vi "CreateChannel.vi"(0 "task in":refnum<class "WaveformTask.lvclass">, 5 "Chan Name Array":string[](array[string]), 9 "instance":u8, 11 "error in":errorcluster) -> (4 "Task out":refnum<class "WaveformTask.lvclass">, 15 "error out":errorcluster)   [LabVIEW 2017, in "WaveformTask.lvclass"]
uses:
  WaveformTask.lvclass
  WaveformTask.lvclass/WaveformTask.ctl
  <instrlib>/_niInstr/FIFO Register Bus/v1/Host/niInstr FIFO Register Bus v1 Host.lvclass
  C:/Program Files (x86)/National Instruments/LabVIEW 2017/instr.lib/_niInstr/Instruction Framework/v1/Host/Instruction Target/niInstr Instruction Target v1 Host.lvclass
  <instrlib>/_niInstr/Instruction Framework/v1/Host/Subsystem Map/Private/Lookup Single Context.vi
  <instrlib>/_niInstr/Instruction Framework/v1/Host/Subsystem Map/niInstr Subsystem Map v1 Host.lvclass
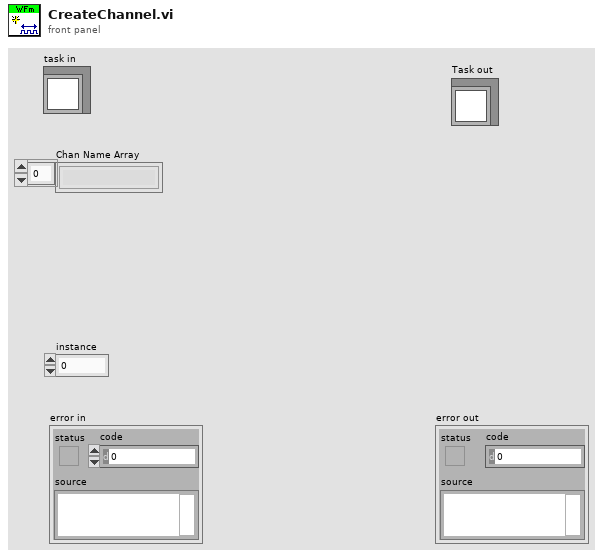
[diagram p1: front panel]
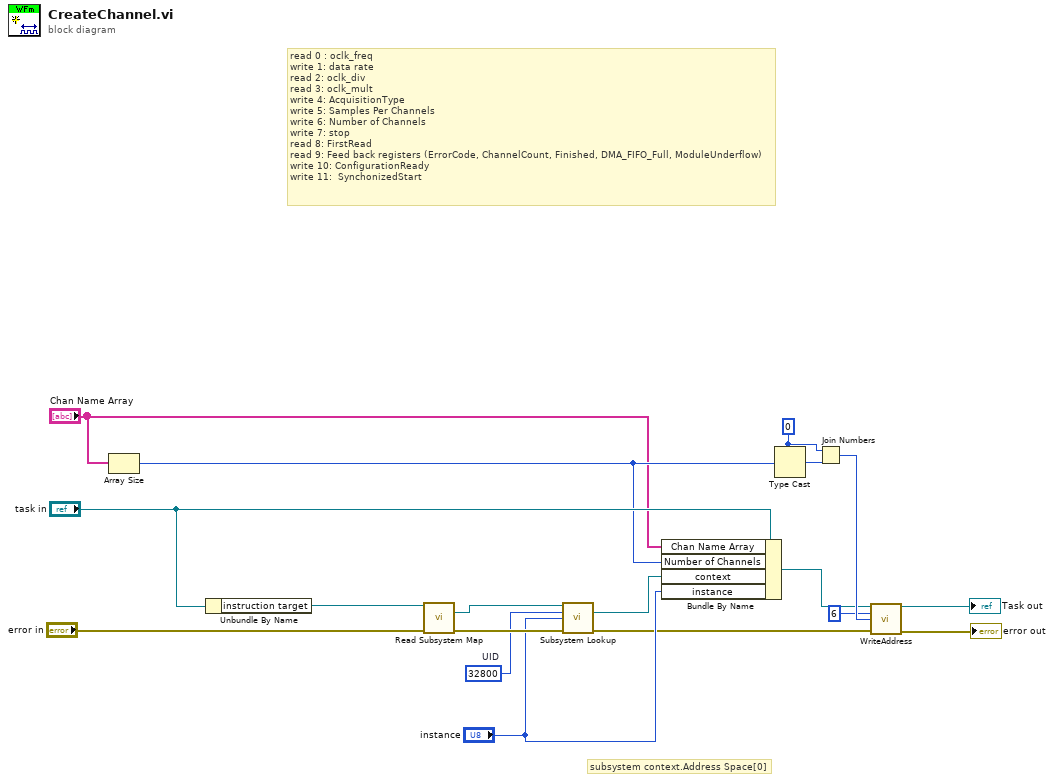
[diagram p0: block diagram]
diagram:
  w14 = u32 0
  w16 = u16 32800  # UID
  # "subsystem context.Address Space[0]"
  # "read 0 : oclk_freq\nwrite 1: data rate\nread 2: oclk_div\nread 3: oclk_mult\nwrite 4: AcquisitionType\nwrite 5: Samples Per Channels\nwrite 6: Number of Channels\nwrite 7: stop\nread 8: FirstRead\nread 9: Feed back registers (ErrorCode, ChannelCount, Finished, DMA_FIFO_Full, ModuleUnderflow)\nwrite 10: ConfigurationReady\nwrite 11:  SynchonizedStart"
  n1 = Array Size(array="Chan Name Array") -> (size(s)=w2:i32)
  n2 = Unbundle By Name("task in") -> ("instruction target"=w8:refnum<class "niInstr FIFO Register Bus v1 Host.lvclass">)
  n3 = call <instrlib>:"Read Subsystem Map.vi"("instruction target in"=w8, "error in"="error in") -> ("subsystem map"=w17:refnum<class "niInstr Subsystem Map v1 Host.lvclass">, "error out"=w18:errorcluster)  [unwired: 11 in, 1 out]
  n4 = call-poly <instrlib>:"Subsystem Lookup.vi"("subsystem map in"=w17, "UID"=w16, "instance"="instance", "error in"=w18) -> ("context"=w6:refnum<class "niInstr Instruction Framework Context v1 Host.lvclass">, "error out"=w3:errorcluster)  [unwired: 8 in, 2 out]
  n5 = Bundle By Name(cluster="task in", "Chan Name Array"="Chan Name Array", "Number of Channels"=w2, "context"=w6, "instance"="instance") -> (w4:refnum<class "WaveformTask.lvclass">)
  n6 = Type Cast(type=w14, x=w2) -> (*(type *) &x=w15:u32)
  n7 = Join Numbers(hi=w14, lo=w15) -> ((hi.lo)=w12:u64)
  n8 = call "WriteAddress.vi"("Task in"=w4, "address"=u64 6, "data"=w12, "error in (no error)"=w3) -> ("Task out"=→"Task out":refnum<class "WaveformTask.lvclass">, "error out"=→"error out":errorcluster)  [unwired: 10 in]
